vi "d(f2+g2u)_dx3.vi"(1 "x3_":dbl, 4 "x4_":dbl, 6 "F":dbl) -> (23 "d(f2+g2u)/dx3":dbl)   [LabVIEW 2014]
uses:
  <vilib>/Simulation/Implementation/Shared/SIMSCR Execution Mode.ctl
  <vilib>/Simulation/Scripting/Companion Diagram/SimConfigNode/SimParams.ctl
  <vilib>/Simulation/Scripting/Companion Diagram/SimConfigNode/_simSolvers.ctl
  <vilib>/Simulation/Param Hierarchy/Typedefs/SIMPH Param Control Actions.ctl
  <vilib>/Simulation/Implementation/Shared/NILVSim_ParamChanged.vi
  <vilib>/Simulation/Implementation/Shared/NILVSIM_BeginStep.vi
  <vilib>/Simulation/SignalArithmetic/Implementation/NILVSim Gain.llb/SIM Gain (scalar).vi
  <vilib>/Simulation/Implementation/Shared/NILVSim_Manager.vi
  <vilib>/Utility/error.llb/Clear Errors.vi
  <vilib>/Simulation/Implementation/Shared/NILVSim_FinalizeModel.vi
  <vilib>/Simulation/Implementation/Shared/SIM Unbundle Sim Info.vi
  <vilib>/Simulation/Implementation/Shared/SIMSH Read Queue.vi
  <vilib>/Simulation/Implementation/Shared/NILVSim_Initialize.vi
  <vilib>/Simulation/Utility/Implementation/NILVSim Get Time and IsAcceptedStep.vi
  <vilib>/Simulation/Implementation/Shared/NILVSim_GetModelError.vi
  <vilib>/Simulation/Implementation/Shared/SIM SimErrorHandler.vi
  <vilib>/Simulation/Implementation/Shared/SIM Bundle Sim Info.vi
  <vilib>/Simulation/Scripting/Companion Diagram/SimConfigNode/SimDog.xnode
  <vilib>/Simulation/Implementation/XNodeFramework/SimXNode/SimX.xnode
  <vilib>/Simulation/Implementation/Shared/NI_SIM_Implementation.lvlib
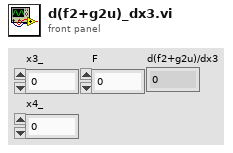
[diagram p1: front panel]
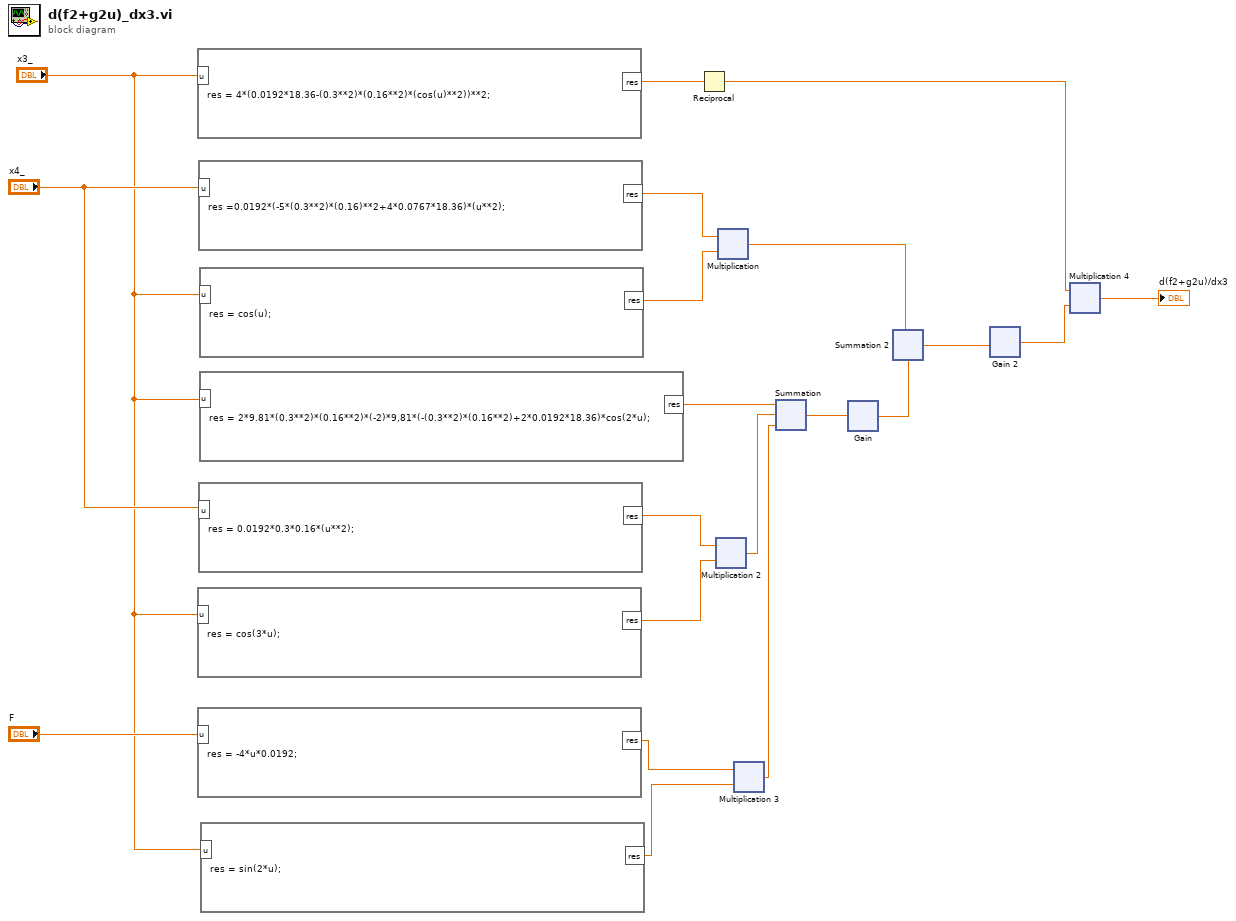
[diagram p0: block diagram]
diagram:
  n1 = formula code="res = 4*(0.0192*18.36-(0.3**2)*(0.16**2)*(cos(u)**2))**2;" ("Formelknoten")("u"="x3_") -> ("res"=w20:dbl)
  n2 = formula code="res = cos(3*u);" ("Formelknoten 5")("u"="x3_") -> ("res"=w13:dbl)
  n3 = formula code="res = -4*u*0.0192;" ("Formelknoten 7")("u"="F") -> ("res"=w10:dbl)
  n4 = formula code="res =0.0192*(-5*(0.3**2)*(0.16)**2+4*0.0767*18.36)*(u**2);" ("Formelknoten 2")("u"="x4_") -> ("res"=w19:dbl)
  n5 = formula code="res = 0.0192*0.3*0.16*(u**2);" ("Formelknoten 6")("u"="x4_") -> ("res"=w14:dbl)
  n6 = formula code="res = cos(u);" ("Formelknoten 3")("u"="x3_") -> ("res"=w18:dbl)
  n7 = formula code="res = 2*9.81*(0.3**2)*(0.16**2)*(-2)*9,81*(-(0.3**2)*(0.16**2)+2*0.0192*18.36)*cos(2*u);" ("Formelknoten 4")("u"="x3_") -> ("res"=w17:dbl)
  n8 = formula code="res = sin(2*u);" ("Formelknoten 8")("u"="x3_") -> ("res"=w9:dbl)
  n9 = Reciprocal ("Kehrwert")(x=w20) -> (1/x=w2:dbl)
  n10 = xnode ("Multiplication 2")("Operand1"=w14, "Operand2"=w13) -> ("Result"=w12:dbl)
  n11 = xnode ("Multiplication")("Operand1"=w19, "Operand2"=w18) -> ("Result"=w5:dbl)
  n12 = xnode ("Multiplication 3")("Operand1"=w10, "Operand2"=w9) -> ("Result"=w8:dbl)
  n13 = xnode ("Summation")("Operand1"=w17, "Operand2"=w12, "Operand3"=w8) -> ("Result"=w7:dbl)
  n14 = xnode "Gain"("input"=w7) -> ("output"=w6:dbl)  [unwired: 3 in]
  n15 = xnode ("Summation 2")("Operand1"=w5, "Operand2"=w6) -> ("Result"=w4:dbl)
  n16 = xnode "Gain 2"("input"=w4) -> ("output"=w3:dbl)  [unwired: 3 in]
  n17 = xnode ("Multiplication 4")("Operand1"=w2, "Operand2"=w3) -> ("Result"=→"d(f2+g2u)/dx3":dbl)
